vi "logTof.vi"(8 "ToF Reading":T1, 9 "Index":i32) -> ()   [LabVIEW 2017]
uses:
  Type Defs/tofReading.ctl
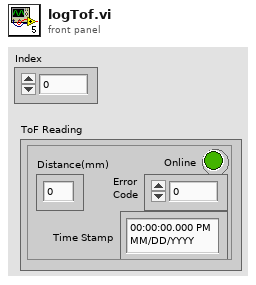
[diagram p1: front panel]
types:
  T1 = typedef "tofReading.ctl" = cluster{"Distance(mm)":u8, "Online":bool, "Error\nCode":u8, "Time Stamp":timestamp}
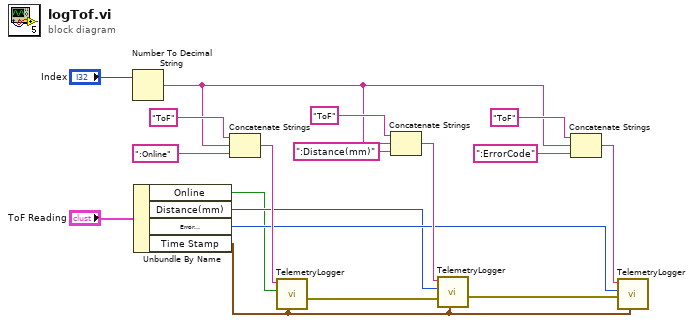
[diagram p0: block diagram]
diagram:
  n1 = Number To Decimal String(number="Index") -> (decimal integer string=w8:string)  [unwired: 1 in]
  n2 = Unbundle By Name("ToF Reading") -> ("Online"=w3:bool, "Distance(mm)"=w4:u8, "Error\nCode"=w5:u8, "Time Stamp"=w6:timestamp)
  n3 = Concatenate Strings("ToF", w8, ":Online") -> (w15:string)
  n4 = call "TelemetryLogger.vi"("Time Stamp"=w6, "Data"=w3, "Sensor:Reading"=w15) -> ("Error Out"=w2:errorcluster)  [unwired: 8 in]
  n5 = Concatenate Strings("ToF", w8, ":Distance(mm)") -> (w14:string)
  n6 = call "TelemetryLogger.vi"("Time Stamp"=w6, "Error In"=w2, "Data"=w4, "Sensor:Reading"=w14) -> ("Error Out"=w1:errorcluster)  [unwired: 7 in]
  n7 = Concatenate Strings("ToF", w8, ":ErrorCode") -> (w9:string)
  n8 = call "TelemetryLogger.vi"("Time Stamp"=w6, "Error In"=w1, "Data"=w5, "Sensor:Reading"=w9) -> ()  [unwired: 7 in, 1 out]
